vi "DLU with 4 Wire Handshake.vi"(6 "ready for output":bool=TRUE, 9 "Input Valid":bool=TRUE, 10 "Input Data":T3, 11 "Private Data In":T2={"DLU To SPI Engine Data FIFO"="DLU To SPI Engine Data", "SPI Engine to DLU Data FIFO"="SPI Engine to DLU Data", "Data to SPI Engine (Cache) Register"="Data to SPI Engine (Cache)", "SPI PHY Settings to SPI Engine (Cahche) Register"="SPI PHY Settings to SPI Engine (Cache)"}) -> (1 "Output Valid":bool=TRUE, 2 "Output Data":T1, 4 "ready for Input":bool)   [LabVIEW 2014, in "IO Node Logic Template_SPIBus0.lvlib"]
uses:
  IO Node Logic Template_SPIBus0.lvlib
  Node/Controls/Node_Command_Sent.ctl
  <vilib>/SPI API/SPIAPI/Controls/Internal Data (SPI API).ctl
  <vilib>/SPI API/SPIAPI/Controls/SPI Response Information.ctl
  <instrlib>/_niInstr/Basic Elements/v1/FPGA/Private/Count Up U16.vi
  <instrlib>/_niInstr/Basic Elements/v1/FPGA/niInstr Basic Elements v1 FPGA.lvlib
panel:
  out "count out 3":u16
  out "count out 2":u16
  out "count out":u16
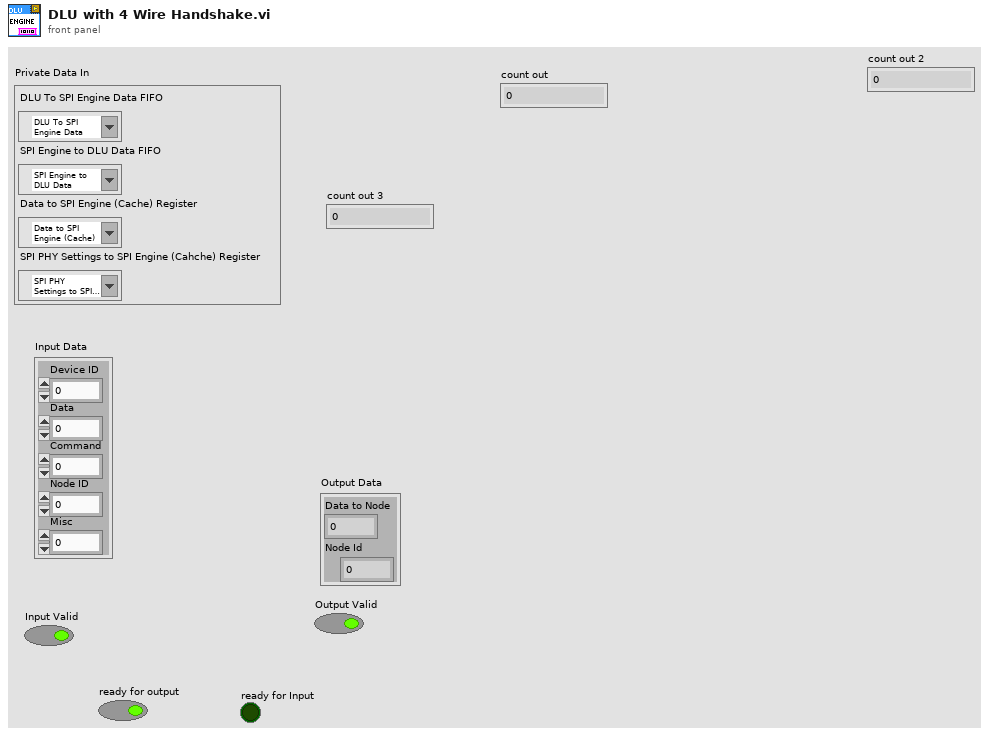
[diagram p1: front panel]
types:
  T1 = typedef "SPI Response Information.ctl" = cluster{"Data to Node":u64, "Node Id":u16}
  T2 = typedef "Internal Data (SPI API).ctl" = cluster{"DLU To SPI Engine Data FIFO":refnum<k21>, "SPI Engine to DLU Data FIFO":refnum<k21>, "Data to SPI Engine (Cache) Register":refnum<k21>, "SPI PHY Settings to SPI Engine (Cahche) Register":refnum<k21>}
  T3 = typedef "IO Node Logic Template_SPIBus0.lvlib/Node_Command_Sent.ctl" = cluster{"Device ID":u8, "Data":u64, "Command":u8, "Node ID":u8, "Misc":u8}
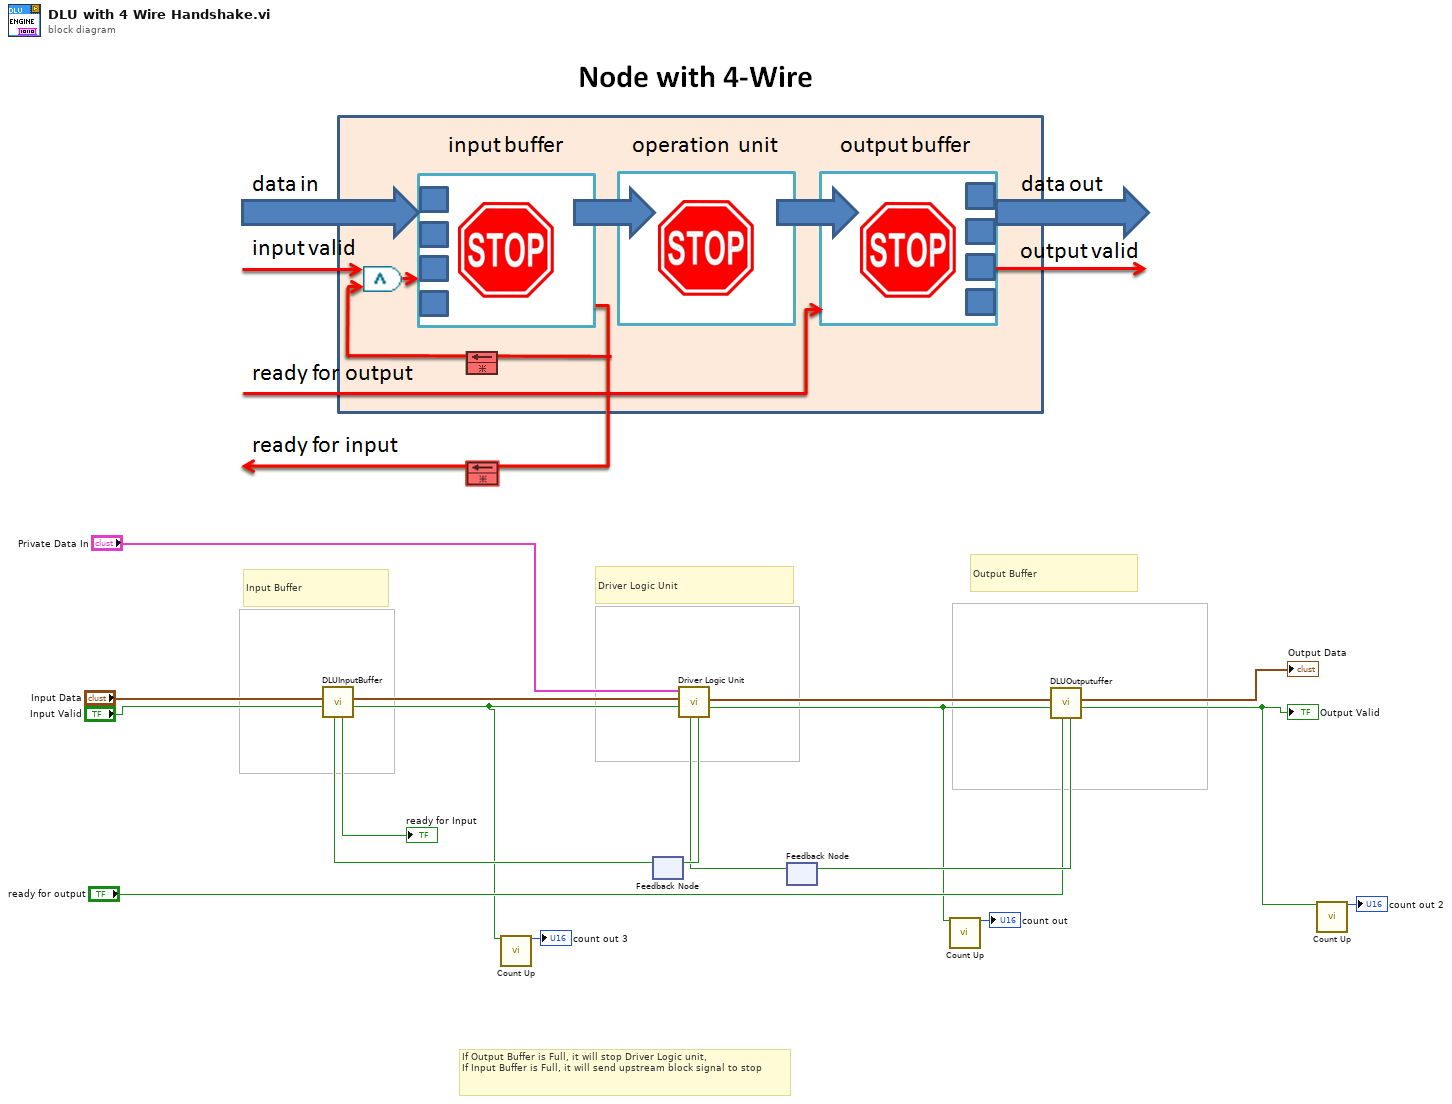
[diagram p0: block diagram]
diagram:
  # "If Output Buffer is Full, it will stop Driver Logic unit,\nIf Input Buffer is Full, it will send upstream block signal to stop"
  # "Input Buffer"
  # "Output Buffer"
  # "Driver Logic Unit"
  n1 = feedback #1() -> (w10:bool)  [unwired: 1 in]
  n2 = call "DLUInputBuffer.vi"("Ready for Output"=w10, "Input Valid"="Input Valid", "Input Data"="Input Data") -> (1:"Output Data"=w1:bool, 2:"Output Data"=w17:T3, "Ready For Input"=→"ready for Input":bool)  [unwired: 6 in]
  n3 = call-poly <instrlib>:"Count Up.vi"("increment"=w1) -> ("count out"=→"count out 3":u16)  [unwired: 14 in]
  n4 = feedback #2() -> (w11:bool)  [unwired: 1 in]
  n5 = call "Driver Logic Unit.vi"("Ready for Output"=w11, "New Cmd Valid?"=w1, "Command sent by Node"=w17, "Private Data In"="Private Data In") -> ("SPI Data Valid?"=w6:bool, "SPI Bus Read Data"=w8:T1, "Ready For Input?"=w18:bool)  [unwired: 4 in, 1 out]
  n6 = feedback-in #1(w18) -> ()
  n7 = call-poly <instrlib>:"Count Up.vi"("increment"=w6) -> ("count out"=→"count out":u16)  [unwired: 14 in]
  n8 = call "DLUOutputuffer.vi"("Ready for Output"="ready for output", "Input Valid"=w6, "Input Data"=w8) -> ("Output Valid"=w3:bool, "Output Data"=→"Output Data":cluster{"Data to Node":u64, "Node Id":u16}, "Ready For Input"=w13:bool)  [unwired: 6 in]
  "Output Valid" <- w3
  n9 = feedback-in #2(w13) -> ()
  n10 = call-poly <instrlib>:"Count Up.vi"("increment"=w3) -> ("count out"=→"count out 2":u16)  [unwired: 14 in]
